vi "进程信息Lv2.vi"(4 "error in (no error)":errorcluster, 5 "状态":string, 6 "进程状态":refnum<vi>, 7 "显示？":bool) -> (0 "error out":errorcluster)   [LabVIEW 2016]
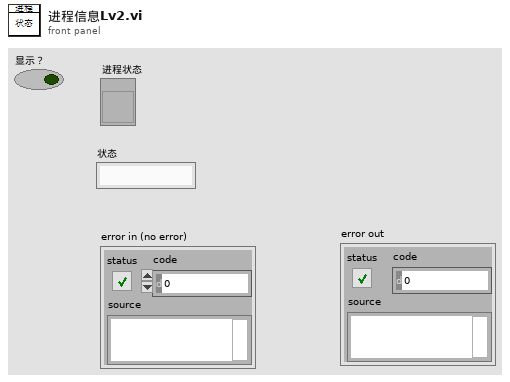
[diagram p1: front panel]
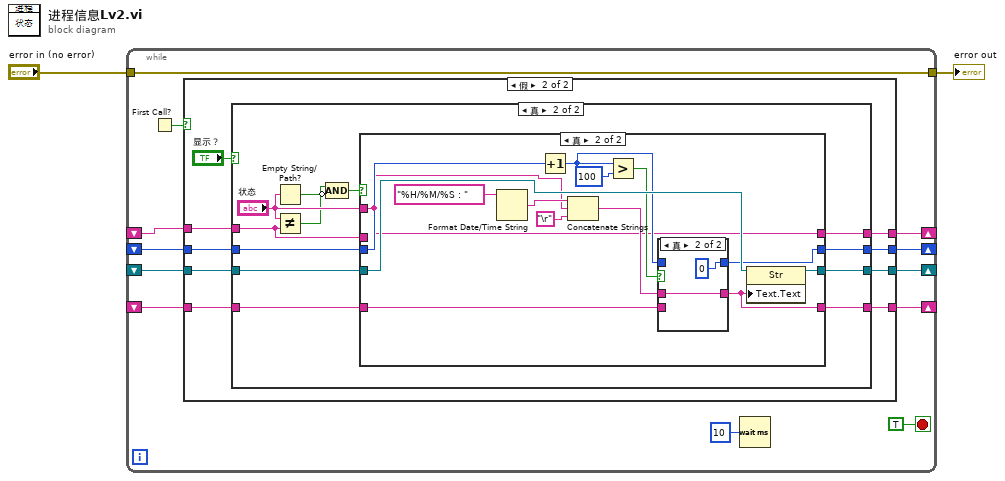
[diagram p0: block diagram]
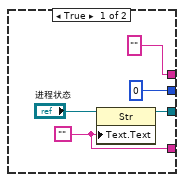
[diagram p2: hidden frame]
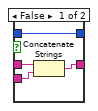
[diagram p5: hidden frame]
diagram:
  n1 = while {
    shift-right: [w10] -> _
    shift-left: _ -> [w12]
    tunnel: "error in (no error)" -> [w9]
    tunnel: [w9] -> w1
    shift-right: [w13] -> _
    shift-left: _ -> [w11]
    shift-right: [w8] -> _
    shift-left: _ -> [w7]
    shift-right: [w6] -> _
    shift-left: _ -> [w5]
    stop <- TRUE stop-if-true
    n2 = First Call?() -> (First Call?: T/F=w4:bool)
    n3 = case shown="假" w4 {
      tunnel: [w19 w27] -> w13
      tunnel: w12 -> [_ w28]
      tunnel: w11 -> [_ w23]
      tunnel: [w18 w26] -> w10
      tunnel: [0 w25] -> w8
      tunnel: w7 -> [_ w24]
      tunnel: ["" ("状态") w22] -> w6
      tunnel: w5 -> [_ w21]
      frame True {
        w19 = ""
        n4 = property class="Str"(reference="进程状态", "Text.Text"=w19) -> (reference out=w18:refnum<vi>)  [unwired: 1 in, 1 out]
      }
      frame False {
        n5 = case shown="真" "显示？" {
          tunnel: w28 -> [w30 w44]
          tunnel: [w29 w43] -> w27
          tunnel: [w30 w42] -> w26
          tunnel: [w31 w41] -> w25
          tunnel: w24 -> [w31 w40]
          tunnel: w23 -> [w29 w39]
          tunnel: [w32 w38] -> w22
          tunnel: w21 -> [w32 w37]
          frame False {
          }
          frame True {
            n6 = Empty String/Path?(string/path="状态") -> (empty?=w33:bool)
            n7 = Not Equal?(x="状态", y=w37) -> (x != y?=w35:bool)
            n8 = Compound Arithmetic op=AND ("复合运算")(w35, invert w33) -> (w34:bool)
            n9 = case shown="真" w34 {
              tunnel: w44 -> [w48 w62]
              tunnel: [w47 w61] -> w43
              tunnel: [w48 w60] -> w42
              tunnel: [w46 w54] -> w41
              tunnel: w40 -> [w46 w53]
              tunnel: w39 -> [w47 w50]
              tunnel: "状态" -> [_ w49]
              tunnel: [w45 w49] -> w38
              tunnel: w37 -> [w45 _]
              frame False {
              }
              frame True {
                n10 = Format Date/Time String(time format string (%c)="%H/%M/%S : ") -> (date/time string=w58:string)  [unwired: 2 in]
                n11 = Increment(x=w53) -> (x+1=w55:i32)
                n12 = Concatenate Strings(w58, w49, "\r") -> (w51:string)
                n13 = Greater?(x=w55, y=100) -> (0:w56:bool)
                n14 = case shown="真" w56 {
                  tunnel: w51 -> [w64 w68]
                  tunnel: [w66 w68] -> w61
                  tunnel: w50 -> [w65 _]
                  tunnel: w55 -> [w63 _]
                  tunnel: [w63 0] -> w54
                  frame False {
                    n15 = Concatenate Strings(w64, w65) -> (w66:string)
                  }
                  frame True {
                  }
                }
                n16 = property class="Str"(reference=w62, "Text.Text"=w61) -> (reference out=w60:refnum<vi>)  [unwired: 1 in, 1 out]
              }
            }
          }
        }
      }
    }
    n17 = Wait (ms)(milliseconds to wait=u32 10 ("等待时间（毫秒）")) -> ()  [unwired: 1 out]
  }
  "error out" <- w1
